vi "RGB2GRAY.vi"(3 "B":u8, 4 "G":u8, 5 "R":u8) -> (0 "gray B":u8, 1 "gray G":u8, 2 "gray R":u8)   [LabVIEW 2020]
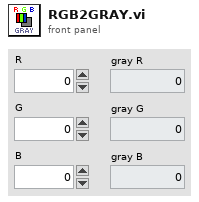
[diagram p1: front panel]
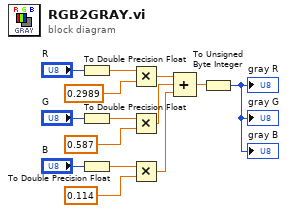
[diagram p0: block diagram]
diagram:
  n1 = To Double Precision Float(number="R") -> (double precision float=w11:dbl)
  n2 = To Double Precision Float(number="G") -> (double precision float=w9:dbl)
  n3 = To Double Precision Float(number="B") -> (double precision float=w7:dbl)
  n4 = Multiply(x=w11, y=0.2989) -> (x*y=w5:dbl)
  n5 = Multiply(x=w9, y=0.587) -> (x*y=w4:dbl)
  n6 = Multiply(x=w7, y=0.114) -> (x*y=w3:dbl)
  n7 = Compound Arithmetic op=ADD(w5, w4, w3) -> (w2:dbl)
  n8 = To Unsigned Byte Integer(number=w2) -> (unsigned 8bit integer=→"gray R" →"gray G" →"gray B":u8)
